vi "LCB Get Device Property.vi"(7 "Property ID":i32, 8 "error in (no error)":errorcluster caption="Fehler (Eingang, kein Fehler)", 11 "Device Handle":i64) -> (0 "error out":errorcluster caption="Fehler (Ausgang)", 3 "Property Value":dbl)   [LabVIEW 2021, in "labbCAN_Bus_API.lvlib"]
doc: "LCB_Func long __stdcall LCB_GetNodeId(dev_hdl hDev_in);"
uses:
  labbCAN_Bus_API.lvlib
  labbCAN_Bus_API.dll
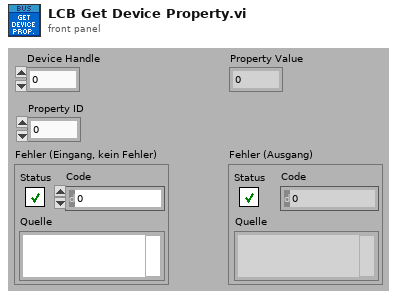
[diagram p1: front panel]
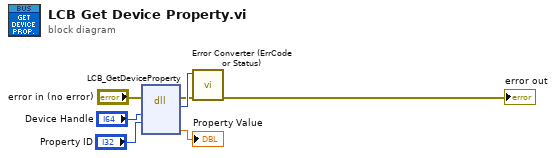
[diagram p0: block diagram]
diagram:
  n1 = dll-call lib="C:/Users/olaja/AppData/Local/CETONI_SDK/labbCAN_Bus_API.*" fn="LCB_GetDeviceProperty"(error in="error in (no error)", "DeviceHandle"="Device Handle", "PropertyId"="Property ID") -> (error out=w4:errorcluster, "Rückgabetyp"=w7:i32, "Value"=→"Property Value":dbl)  [unwired: 5 in, 1 out]
  n2 = call "Error Converter (ErrCode or Status).vi"("error in (no error)"=w4, "error code"=w7) -> ("error out"=→"error out":errorcluster)  [unwired: 9 in]
